vi "Command Window (LAN).vi"() -> ()   [LabVIEW 2011]
panel:
  in  "Query":bool
  in  "abort (F)":bool
  in  "address":string
  out "connection ID out":refnum<k5>
  out "data out":string
  in  "data in":string
  out "error out":errorcluster
  in  "error in (no error)":errorcluster
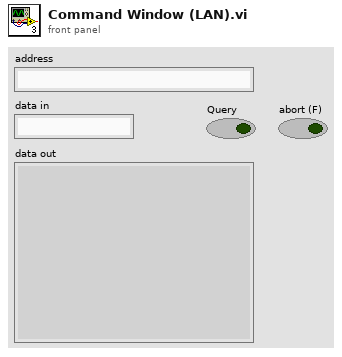
[diagram p1: front panel]
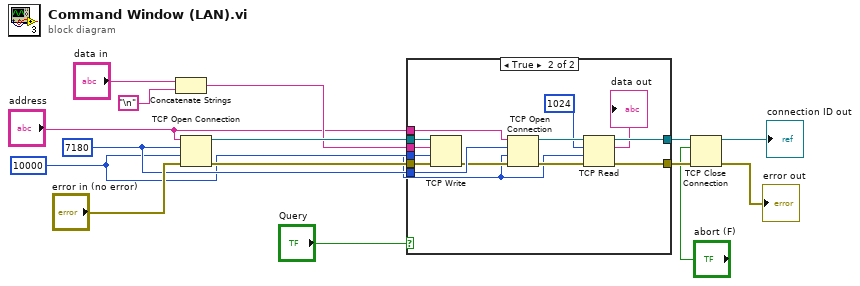
[diagram p0: block diagram]
diagram:
  w3 = 10000 ("timeout ms (60000)")
  w4 = u16 7180 ("remote port or service name")
  n1 = Concatenate Strings("data in", "\n") -> (w8:string)
  n2 = TCP Open Connection(address="address", remote port or service name=w4, timeout ms (60000)=w3, error in (no error)="error in (no error)") -> (connection ID=w12:refnum<k5>, error out=w14:errorcluster)  [unwired: 1 in]
  n3 = case shown="True" "Query" {
    tunnel: w14 -> [w16 w30]
    tunnel: [w16 w29] -> w13
    tunnel: w12 -> [w17 w28]
    tunnel: [w17 w27] -> w11
    tunnel: w8 -> [_ w25]
    tunnel: "address" -> [_ w24]
    tunnel: w4 -> [_ w23]
    tunnel: w3 -> [_ w18]
    frame False {
    }
    frame True {
      n4 = TCP Write(connection ID=w28, data in=w25, error in (no error)=w30, 9:w18) -> (error out=w22:errorcluster)  [unwired: 2 out]
      n5 = TCP Open Connection(address=w24, remote port or service name=w23, timeout ms (60000)=w18, error in (no error)=w22) -> (connection ID=w20:refnum<k5>, error out=w21:errorcluster)  [unwired: 1 in]
      n6 = TCP Read(connection ID=w20, bytes to read=1024, error in (no error)=w21, 9:w18) -> (connection ID out=w27:refnum<k5>, data out=→"data out":string, error out=w29:errorcluster)  [unwired: 1 in]
    }
  }
  n7 = TCP Close Connection(connection ID=w11, abort (F)="abort (F)", error in (no error)=w13) -> (connection ID out=→"connection ID out":refnum<k5>, error out=→"error out":errorcluster)
